vi "Write DG.vi"(8 "error in (no error)":errorcluster, 10 "BME_DG_Base":refnum<class "BME_DG_Base.lvclass">, 11 "BME_DG_System in":refnum<class "BME_DG_System.lvclass">) -> (0 "error out":errorcluster, 3 "BME_DG_System out":refnum<class "BME_DG_System.lvclass">)   [LabVIEW 2009, in "POLARIS BME DG.lvlib" / "BME_DG_System.lvclass"]
uses:
  BME_DG_System.lvclass
  BME_DG_Base/BME_DG_Base.lvclass
  BME_DG_System.lvclass/BME_DG_System.ctl
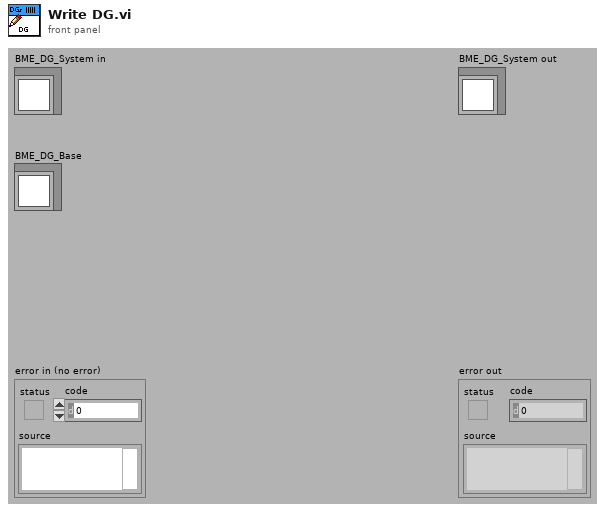
[diagram p1: front panel]
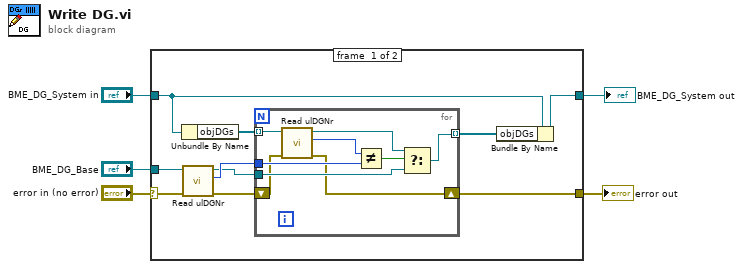
[diagram p0: block diagram]
diagram:
  n1 = case shown="No Error" "error in (no error)" {
    selector: "error in (no error)" -> [w8 w26]
    tunnel: [w6 w26] -> w4
    tunnel: [w10 w25] -> w2
    tunnel: "BME_DG_System in" -> [w15 w25]
    tunnel: "BME_DG_Base" -> [w13 _]
    frame #0 {
      n2 = Unbundle By Name(w15) -> ("objDGs"=w14:refnum<class "BME_DG_Base.lvclass">[])
      n3 = call-dynamic "Read ulDGNr.vi"("error in (no error)"=w8, "BME_DG_Base in"=w13) -> ("error out"=w7:errorcluster, "ulDGNr"=w12:u32, "BME_DG_Base out"=w11:refnum<class "BME_DG_Base.lvclass">)  [unwired: 6 in, 1 out]
      n4 = for {
        tunnel: w14 -> [w24] mode=indexing
        tunnel: w12 -> [w22]
        tunnel: w11 -> [w19]
        tunnel: [w18] -> w9 mode=indexing
        shift-right: [w16] -> w6
        shift-left: w7 -> [w17]
        n5 = call-dynamic "Read ulDGNr.vi"("error in (no error)"=w17, "BME_DG_Base in"=w24) -> ("error out"=w16:errorcluster, "ulDGNr"=w23:u32, "BME_DG_Base out"=w20:refnum<class "BME_DG_Base.lvclass">)  [unwired: 6 in, 1 out]
        n6 = Not Equal?(x=w23, y=w22) -> (x != y?=w21:bool)
        n7 = Select(t=w20, s=w21, f=w19) -> (s? t:f=w18:refnum<class "BME_DG_Base.lvclass">)
      }
      n8 = Bundle By Name(cluster=w15, "objDGs"=w9) -> (w10:refnum<class "BME_DG_System.lvclass">)
    }
    frame #1 {
    }
  }
  "error out" <- w4
  "BME_DG_System out" <- w2
